vi "MTM2_getSample_rawTelemetry.vi"(8 "error in (no error)":errorcluster, 11 "rawTelemetry_Ctl":T1) -> (0 "error out":errorcluster, 2 "function return":i32, 3 "rawTelemetry_Ctl out":T1)   [LabVIEW 2018, in "SALLV_MTM2.lvlib"]
doc: "int MTM2_shm_getSample_rawTelemetryLV(MTM2_rawTelemetryLV *rawTelemetry_Ctl );"
uses:
  SALLV_MTM2.lvlib
  DataTypes/rawTelemetry.ctl
  SALLV_MTM2.so
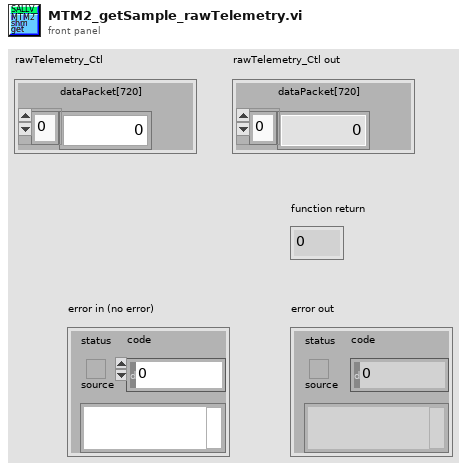
[diagram p1: front panel]
types:
  T1 = typedef "SALLV_MTM2.lvlib/rawTelemetry.ctl" = cluster{"dataPacket[720]":i32[]}
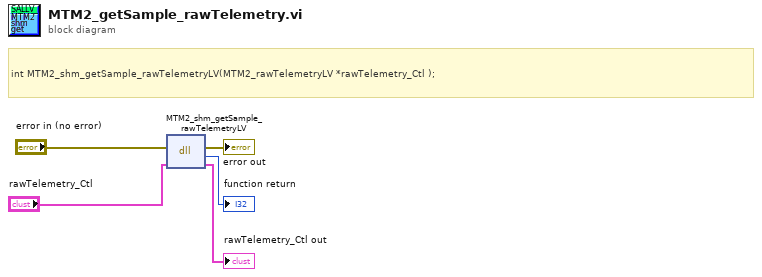
[diagram p0: block diagram]
diagram:
  # "int MTM2_shm_getSample_rawTelemetryLV(MTM2_rawTelemetryLV *rawTelemetry_Ctl );"
  n1 = dll-call lib="home/ttsai/Document/salApiMTM2/SALLV_MTM2/SALLV_MTM2.*" fn="MTM2_shm_getSample_rawTelemetryLV"(error in="error in (no error)", "rawTelemetry_Ctl"="rawTelemetry_Ctl") -> (error out=→"error out":errorcluster, →"function return":i32, "rawTelemetry_Ctl"=→"rawTelemetry_Ctl out":T1)  [unwired: 2 in, 1 out]
